vi "example_02_convert.vi"() -> ()   [LabVIEW 2015, in "lv-unit-conversion.lvlib"] (continued)
, "dimension"="M/L3", "is_si_unit"=TRUE, "category"="derived", "base_unit"="kg/m3", "conversion_reference"="DERIVED", "is_exact"=TRUE, "a"=0.0, "b"=0.45359237, "c"=158.987294928, "d"=0.0, "underlying_def"="", "description"=""}, {"symbol"="0.001 lbm/gal[UK]", "name"="pound-mass per thousand UK gallon", "dimension"="M/L3", "is_si_unit"=TRUE, "category"="derived", "base_unit"="kg/m3", "conversion_reference"="DERIVED", "is_exact"=TRUE, "a"=0.0, "b"=0.45359237, "c"=4.54609, "d"=0.0, "underlying_def"="", "description"=""}, {"symbol"="0.001 lbm/gal[US]", "name"="pound-mass per thousand US gallon", "dimension"="M/L3", "is_si_unit"=TRUE, "category"="derived", "base_unit"="kg/m3", "conversion_reference"="DERIVED", "is_exact"=TRUE, "a"=0.0, "b"=0.45359237, "c"=3.785411784, "d"=0.0, "underlying_def"="", "description"=""}, {"symbol"="0.01 grain/ft3", "name"="grain per hundred cubic foot", "dimension"="M/L3", "is_si_unit"=TRUE, "category"="derived", "base_unit"="kg/m3", "conversion_reference"="DERIVED", "is_exact"=TRUE, "a"=0.0, "b"=6.479891e-05, "c"=2.8316846592, "d"=0.0, "underlying_def"="", "description"=""}, {"symbol"="0.1 lbm/bbl", "name"="pound-mass per ten barrel", "dimension"="M/L3", "is_si_unit"=TRUE, "category"="derived", "base_unit"="kg/m3", "conversion_reference"="DERIVED", "is_exact"=TRUE, "a"=0.0, "b"=0.45359237, "c"=1.58987294928, "d"=0.0, "underlying_def"="", "description"=""}, {"symbol"="10 Mg/m3", "name"="ten thousand kilogram per cubic metre", "dimension"="M/L3", "is_si_unit"=TRUE, "category"="derived", "base_unit"="kg/m3", "conversion_reference"="DERIVED", "is_exact"=TRUE, "a"=0.0, "b"=10000.0, "c"=1.0, "d"=0.0, "underlying_def"="", "description"=""}, {"symbol"="g/cm3", "name"="gram per cubic centimetre", "dimension"="M/L3", "is_si_unit"=TRUE, "category"="derived", "base_unit"="kg/m3", "conversion_reference"="DERIVED", "is_exact"=TRUE, "a"=0.0, "b"=1000.0, "c"=1.0, "d"=0.0, "underlying_def"="", "description"=""}, {"symbol"="g/dm3", "name"="gram per cubic decimetre", "dimension"="M/L3", "is_si_unit"=TRUE, "category"="derived", "base_unit"="kg/m3", "conversion_reference"="DERIVED", "is_exact"=TRUE, "a"=0.0, "b"=1.0, "c"=1.0, "d"=0.0, "underlying_def"="", "description"=""}, {"symbol"="g/gal[UK]", "name"="gram per UK gallon", "dimension"="M/L3", "is_si_unit"=TRUE, "category"="derived", "base_unit"="kg/m3", "conversion_reference"="DERIVED", "is_exact"=TRUE, "a"=0.0, "b"=0.001, "c"=0.00454609, "d"=0.0, "underlying_def"="", "description"=""}, {"symbol"="g/gal[US]", "name"="gram per US gallon", "dimension"="M/L3", "is_si_unit"=TRUE, "category"="derived", "base_unit"="kg/m3", "conversion_reference"="DERIVED", "is_exact"=TRUE, "a"=0.0, "b"=0.001, "c"=0.003785411784, "d"=0.0, "underlying_def"="", "description"=""}, {"symbol"="g/L", "name"="gram per litre", "dimension"="M/L3", "is_si_unit"=TRUE, "category"="derived", "base_unit"="kg/m3", "conversion_reference"="DERIVED", "is_exact"=TRUE, "a"=0.0, "b"=1.0, "c"=1.0, "d"=0.0, "underlying_def"="", "description"=""}, {"symbol"="g/m3", "name"="gram per cubic metre", "dimension"="M/L3", "is_si_unit"=TRUE, "category"="derived", "base_unit"="kg/m3", "conversion_reference"="DERIVED", "is_exact"=TRUE, "a"=0.0, "b"=0.001, "c"=1.0, "d"=0.0, "underlying_def"="", "description"=""}, {"symbol"="grain/ft3", "name"="grain per cubic foot", "dimension"="M/L3", "is_si_unit"=TRUE, "category"="derived", "base_unit"="kg/m3", "conversion_reference"="DERIVED", "is_exact"=TRUE, "a"=0.0, "b"=6.479891e-05, "c"=0.028316846592, "d"=0.0, "underlying_def"="", "description"=""}, {"symbol"="grain/gal[US]", "name"="grain per US gallon", "dimension"="M/L3", "is_si_unit"=TRUE, "category"="derived", "base_unit"="kg/m3", "conversion_reference"="DERIVED", "is_exact"=TRUE, "a"=0.0, "b"=6.479891e-05, "c"=0.003785411784, "d"=0.0, "underlying_def"="", "description"=""}, {"symbol"="kg/dm3", "name"="kilogram per cubic decimetre", "dimension"="M/L3", "is_si_unit"=TRUE, "category"="derived", "base_unit"="kg/m3", "conversion_reference"="DERIVED", "is_exact"=TRUE, "a"=0.0, "b"=1000.0, "c"=1.0, "d"=0.0, "underlying_def"="", "description"=""}, {"symbol"="kg/L", "name"="kilogram per litre", "dimension"="M/L3", "is_si_unit"=TRUE, "category"="derived", "base_unit"="kg/m3", "conversion_reference"="DERIVED", "is_exact"=TRUE, "a"=0.0, "b"=1000.0, "c"=1.0, "d"=0.0, "underlying_def"="", "description"=""}, {"symbol"="lbm/bbl", "name"="pound-mass per barrel", "dimension"="M/L3", "is_si_unit"=TRUE, "category"="derived", "base_unit"="kg/m3", "conversion_reference"="DERIVED", "is_exact"=TRUE, "a"=0.0, "b"=0.45359237, "c"=0.158987294928, "d"=0.0, "underlying_def"="", "description"=""}, {"symbol"="lbm/ft3", "name"="pound-mass per cubic foot", "dimension"="M/L3", "is_si_unit"=TRUE, "category"="derived", "base_unit"="kg/m3", "conversion_reference"="DERIVED", "is_exact"=TRUE, "a"=0.0, "b"=0.45359237, "c"=0.028316846592, "d"=0.0, "underlying_def"="", "description"=""}, {"symbol"="lbm/gal[UK]", "name"="pound-mass per UK gallon", "dimension"="M/L3", "is_si_unit"=TRUE, "category"="derived", "base_unit"="kg/m3", "conversion_reference"="DERIVED", "is_exact"=TRUE, "a"=0.0, "b"=0.45359237, "c"=0.00454609, "d"=0.0, "underlying_def"="", "description"=""}, {"symbol"="lbm/gal[US]", "name"="pound-mass per US gallon", "dimension"="M/L3", "is_si_unit"=TRUE, "category"="derived", "base_unit"="kg/m3", "conversion_reference"="DERIVED", "is_exact"=TRUE, "a"=0.0, "b"=0.45359237, "c"=0.003785411784, "d"=0.0, "underlying_def"="", "description"=""}, {"symbol"="lbm/in3", "name"="pound-mass per cubic inch", "dimension"="M/L3", "is_si_unit"=TRUE, "category"="derived", "base_unit"="kg/m3", "conversion_reference"="DERIVED", "is_exact"=TRUE, "a"=0.0, "b"=0.45359237, "c"=1.6387064e-05, "d"=0.0, "underlying_def"="", "description"=""}, {"symbol"="mg/dm3", "name"="milligram per cubic decimetre", "dimension"="M/L3", "is_si_unit"=TRUE, "category"="derived", "base_unit"="kg/m3", "conversion_reference"="DERIVED", "is_exact"=TRUE, "a"=0.0, "b"=0.001, "c"=1.0, "d"=0.0, "underlying_def"="", "description"=""}, {"symbol"="mg/gal[US]", "name"="milligram per US gallon", "dimension"="M/L3", "is_si_unit"=TRUE, "category"="derived", "base_unit"="kg/m3", "conversion_reference"="DERIVED", "is_exact"=TRUE, "a"=0.0, "b"=1e-06, "c"=0.003785411784, "d"=0.0, "underlying_def"="", "description"=""}, {"symbol"="mg/L", "name"="milligram per litre", "dimension"="M/L3", "is_si_unit"=TRUE, "category"="derived", "base_unit"="kg/m3", "conversion_reference"="DERIVED", "is_exact"=TRUE, "a"=0.0, "b"=0.001, "c"=1.0, "d"=0.0, "underlying_def"="", "description"=""}, {"symbol"="Mg/m3", "name"="megagram per cubic metre", "dimension"="M/L3", "is_si_unit"=TRUE, "category"="derived", "base_unit"="kg/m3", "conversion_reference"="DERIVED", "is_exact"=TRUE, "a"=0.0, "b"=1000.0, "c"=1.0, "d"=0.0, "underlying_def"="", "description"=""}, {"symbol"="mg/m3", "name"="milligram per cubic metre", "dimension"="M/L3", "is_si_unit"=TRUE, "category"="derived", "base_unit"="kg/m3", "conversion_reference"="DERIVED", "is_exact"=TRUE, "a"=0.0, "b"=1e-06, "c"=1.0, "d"=0.0, "underlying_def"="", "description"=""}, {"symbol"="t/m3", "name"="tonne per cubic metre", "dimension"="M/L3", "is_si_unit"=TRUE, "category"="derived", "base_unit"="kg/m3", "conversion_reference"="DERIVED", "is_exact"=TRUE, "a"=0.0, "b"=1000.0, "c"=1.0, "d"=0.0, "underlying_def"="", "description"=""}, {"symbol"="ug/cm3", "name"="microgram per cubic centimetre", "dimension"="M/L3", "is_si_unit"=TRUE, "category"="derived", "base_unit"="kg/m3", "conversion_reference"="DERIVED", "is_exact"=TRUE, "a"=0.0, "b"=0.001, "c"=1.0, "d"=0.0, "underlying_def"="", "description"=""}, {"symbol"="kg/m4", "name"="kilogram per metre to the fourth power", "dimension"="M/L4", "is_si_unit"=TRUE, "category"="derived", "base_unit"="", "conversion_reference"="", "is_exact"=FALSE, "a"=0.0, "b"=0.0, "c"=0.0, "d"=0.0, "underlying_def"="", "description"=""}, {"symbol"="g/cm4", "name"="gram per centimetre to the fourth power", "dimension"="M/L4", "is_si_unit"=TRUE, "category"="derived", "base_unit"="kg/m4", "conversion_reference"="DERIVED", "is_exact"=TRUE, "a"=0.0, "b"=100000.0, "c"=1.0, "d"=0.0, "underlying_def"="", "description"=""}, {"symbol"="kg/dm4", "name"="kilogram per decimetre to the fourth power", "dimension"="M/L4", "is_si_unit"=TRUE, "category"="derived", "base_unit"="kg/m4", "conversion_reference"="DERIVED", "is_exact"=TRUE, "a"=0.0, "b"=10000.0, "c"=1.0, "d"=0.0, "underlying_def"="", "description"=""}, {"symbol"="lbm/(gal[UK].ft)", "name"="pound-mass per UK gallon foot", "dimension"="M/L4", "is_si_unit"=TRUE, "category"="derived", "base_unit"="kg/m4", "conversion_reference"="DERIVED", "is_exact"=TRUE, "a"=0.0, "b"=0.45359237, "c"=0.001385648232, "d"=0.0, "underlying_def"="", "description"=""}, {"symbol"="lbm/(gal[US].ft)", "name"="pound-mass per US gallon foot", "dimension"="M/L4", "is_si_unit"=TRUE, "category"="derived", "base_unit"="kg/m4", "conversion_reference"="DERIVED", "is_exact"=TRUE, "a"=0.0, "b"=0.45359237, "c"=0.0011537935117632, "d"=0.0, "underlying_def"="", "description"=""}, {"symbol"="lbm/ft4", "name"="pound-mass per foot to the fourth power", "dimension"="M/L4", "is_si_unit"=TRUE, "category"="derived", "base_unit"="kg/m4", "conversion_reference"="DERIVED", "is_exact"=TRUE, "a"=0.0, "b"=0.45359237, "c"=0.0086309748412416, "d"=0.0, "underlying_def"="", "description"=""}, {"symbol"="Pa.s2/m3", "name"="pascal second squared per cubic metre", "dimension"="M/L4", "is_si_unit"=TRUE, "category"="derived", "base_unit"="kg/m4", "conversion_reference"="DERIVED", "is_exact"=TRUE, "a"=0.0, "b"=1.0, "c"=1.0, "d"=0.0, "underlying_def"="", "description"=""}, {"symbol"="Pa.s/m3", "name"="pascal second per cubic metre", "dimension"="M/L4T", "is_si_unit"=TRUE, "category"="derived", "base_unit"="", "conversion_reference"="", "is_exact"=FALSE, "a"=0.0, "b"=0.0, "c"=0.0, "d"=0.0, "underlying_def"="", "description"=""}, {"symbol"="psi.d/bbl", "name"="psi day per barrel", "dimension"="M/L4T", "is_si_unit"=TRUE, "category"="derived", "base_unit"="Pa.s/m3", "conversion_reference"="DERIVED", "is_exact"=TRUE, "a"=0.0, "b"=384326.3475585072, "c"=0.00010257224319574849, "d"=0.0, "underlying_def"="", "description"=""}, {"symbol"="Pa/m3", "name"="pascal per cubic metre", "dimension"="M/L4T2", "is_si_unit"=TRUE, "category"="derived", "base_unit"="", "conversion_reference"="", "is_exact"=FALSE, "a"=0.0, "b"=0.0, "c"=0.0, "d"=0.0, "underlying_def"="", "description"=""}, {"symbol"="psi2.d/(cP.ft3)", "name"="psi squared day per centipoise cubic foot", "dimension"="M/L4T2", "is_si_unit"=TRUE, "category"="derived", "base_unit"="Pa/m3", "conversion_reference"="DERIVED", "is_exact"=TRUE, "a"=0.0, "b"=1709568766.5238712, "c"=1.1786361425484662e-08, "d"=0.0, "underlying_def"="", "description"=""}, {"symbol"="P", "name"="poise", "dimension"="M/LT", "is_si_unit"=TRUE, "category"="atom", "base_unit"="Pa.s", "conversion_reference"="NIST-SI", "is_exact"=TRUE, "a"=0.0, "b"=0.1, "c"=1.0, "d"=0.0, "underlying_def"="dyne.s/cm2", "description"="The poise is the CGS unit for viscosity (also called dynamic viscosity)."}, {"symbol"="kg/(m.s)", "name"="kilogram per metre second", "dimension"="M/LT", "is_si_unit"=TRUE, "category"="derived", "base_unit"="", "conversion_reference"="", "is_exact"=FALSE, "a"=0.0, "b"=0.0, "c"=0.0, "d"=0.0, "underlying_def"="Pa.s", "description"=""}, {"symbol"="Pa.s", "name"="pascal second", "dimension"="M/LT", "is_si_unit"=TRUE, "category"="derived", "base_unit"="", "conversion_reference"="", "is_exact"=FALSE, "a"=0.0, "b"=0.0, "c"=0.0, "d"=0.0, "underlying_def"="", "description"=""}, {"symbol"="lbm/(ft.h)", "name"="pound-mass per hour foot", "dimension"="M/LT", "is_si_unit"=TRUE, "category"="derived", "base_unit"="kg/(m.s)", "conversion_reference"="DERIVED", "is_exact"=TRUE, "a"=0.0, "b"=0.45359237, "c"=1097.28, "d"=0.0, "underlying_def"="", "description"=""}, {"symbol"="lbm/(ft.s)", "name"="pound-mass per second foot", "dimension"="M/LT", "is_si_unit"=TRUE, "category"="derived", "base_unit"="kg/(m.s)", "conversion_reference"="DERIVED", "is_exact"=TRUE, "a"=0.0, "b"=0.45359237, "c"=0.3048, "d"=0.0, "underlying_def"="", "description"=""}, {"symbol"="dyne.s/cm2", "name"="dyne second per square centimetre", "dimension"="M/LT", "is_si_unit"=TRUE, "category"="derived", "base_unit"="Pa.s", "conversion_reference"="DERIVED", "is_exact"=TRUE, "a"=0.0, "b"=0.1, "c"=1.0, "d"=0.0, "underlying_def"="", "description"=""}, {"symbol"="kgf.s/m2", "name"="thousand gram-force second per square metre", "dimension"="M/LT", "is_si_unit"=TRUE, "category"="derived", "base_unit"="Pa.s", "conversion_reference"="DERIVED", "is_exact"=TRUE, "a"=0.0, "b"=9.80665, "c"=1.0, "d"=0.0, "underlying_def"="", "description"=""}, {"symbol"="lbf.s/ft2", "name"="pound-force second per square foot", "dimension"="M/LT", "is_si_unit"=TRUE, "category"="derived", "base_unit"="Pa.s", "conversion_reference"="DERIVED", "is_exact"=TRUE, "a"=0.0, "b"=4.4482216152605, "c"=0.09290304, "d"=0.0, "underlying_def"="", "description"=""}, {"symbol"="lbf.s/in2", "name"="pound-force second per square inch", "dimension"="M/LT", "is_si_unit"=TRUE, "category"="derived", "base_unit"="Pa.s", "conversion_reference"="DERIVED", "is_exact"=TRUE, "a"=0.0, "b"=4.4482216152605, "c"=0.00064516, "d"=0.0, "underlying_def"="", "description"=""}, {"symbol"="mPa.s", "name"="millipascal second", "dimension"="M/LT", "is_si_unit"=TRUE, "category"="derived", "base_unit"="Pa.s", "conversion_reference"="DERIVED", "is_exact"=TRUE, "a"=0.0, "b"=0.001, "c"=1.0, "d"=0.0, "underlying_def"="", "description"=""}, {"symbol"="N.s/m2", "name"="newton second per square metre", "dimension"="M/LT", "is_si_unit"=TRUE, "category"="derived", "base_unit"="Pa.s", "conversion_reference"="DERIVED", "is_exact"=TRUE, "a"=0.0, "b"=1.0, "c"=1.0, "d"=0.0, "underlying_def"="", "description"=""}, {"symbol"="psi.s", "name"="psi second", "dimension"="M/LT", "is_si_unit"=TRUE, "category"="derived", "base_unit"="Pa.s", "conversion_reference"="DERIVED", "is_exact"=TRUE, "a"=0.0, "b"=4.4482216152605, "c"=0.00064516, "d"=0.0, "underlying_def"="", "description"=""}, {"symbol"="cP", "name"="centipoise", "dimension"="M/LT", "is_si_unit"=TRUE, "category"="prefixed", "base_unit"="Pa.s", "conversion_reference"="DERIVED", "is_exact"=TRUE, "a"=0.0, "b"=0.001, "c"=1.0, "d"=0.0, "underlying_def"="", "description"=""}, {"symbol"="dP", "name"="decipoise", "dimension"="M/LT", "is_si_unit"=TRUE, "category"="prefixed", "base_unit"="Pa.s", "conversion_reference"="DERIVED", "is_exact"=TRUE, "a"=0.0, "b"=0.01, "c"=1.0, "d"=0.0, "underlying_def"="", "description"=""}, {"symbol"="EP", "name"="exapoise", "dimension"="M/LT", "is_si_unit"=TRUE, "category"="prefixed", "base_unit"="Pa.s", "conversion_reference"="DERIVED", "is_exact"=TRUE, "a"=0.0, "b"=1e+17, "c"=1.0, "d"=0.0, "underlying_def"="", "description"=""}, {"symbol"="fP", "name"="femtopoise", "dimension"="M/LT", "is_si_unit"=TRUE, "category"="prefixed", "base_unit"="Pa.s", "conversion_reference"="DERIVED", "is_exact"=TRUE, "a"=0.0, "b"=1e-16, "c"=1.0, "d"=0.0, "underlying_def"="", "description"=""}, {"symbol"="GP", "name"="gigapoise", "dimension"="M/LT", "is_si_unit"=TRUE, "category"="prefixed", "base_unit"="Pa.s", "conversion_reference"="DERIVED", "is_exact"=TRUE, "a"=0.0, "b"=100000000.0, "c"=1.0, "d"=0.0, "underlying_def"="", "description"=""}, {"symbol"="kP", "name"="kilopoise", "dimension"="M/LT", "is_si_unit"=TRUE, "category"="prefixed", "base_unit"="Pa.s", "conversion_reference"="DERIVED", "is_exact"=TRUE, "a"=0.0, "b"=100.0, "c"=1.0, "d"=0.0, "underlying_def"="", "description"=""}, {"symbol"="mP", "name"="millipoise", "dimension"="M/LT", "is_si_unit"=TRUE, "category"="prefixed", "base_unit"="Pa.s", "conversion_reference"="DERIVED", "is_exact"=TRUE, "a"=0.0, "b"=0.0001, "c"=1.0, "d"=0.0, "underlying_def"="", "description"=""}, {"symbol"="MP", "name"="megapoise", "dimension"="M/LT", "is_si_unit"=TRUE, "category"="prefixed", "base_unit"="Pa.s", "conversion_reference"="DERIVED", "is_exact"=TRUE, "a"=0.0, "b"=100000.0, "c"=1.0, "d"=0.0, "underlying_def"="", "description"=""}, {"symbol"="nP", "name"="nanopoise", "dimension"="M/LT", "is_si_unit"=TRUE, "category"="prefixed", "base_unit"="Pa.s", "conversion_reference"="DERIVED", "is_exact"=TRUE, "a"=0.0, "b"=1e-10, "c"=1.0, "d"=0.0, "underlying_def"="", "description"=""}, {"symbol"="pP", "name"="picopoise", "dimension"="M/LT", "is_si_unit"=TRUE, "category"="prefixed", "base_unit"="Pa.s", "conversion_reference"="DERIVED", "is_exact"=TRUE, "a"=0.0, "b"=1e-13, "c"=1.0, "d"=0.0, "underlying_def"="", "description"=""}, {"symbol"="TP", "name"="terapoise", "dimension"="M/LT", "is_si_unit"=TRUE, "category"="prefixed", "base_unit"="Pa.s", "conversion_reference"="DERIVED", "is_exact"=TRUE, "a"=0.0, "b"=100000000000.0, "c"=1.0, "d"=0.0, "underlying_def"="", "description"=""}, {"symbol"="uP", "name"="micropoise", "dimension"="M/LT", "is_si_unit"=TRUE, "category"="prefixed", "base_unit"="Pa.s", "conversion_reference"="DERIVED", "is_exact"=TRUE, "a"=0.0, "b"=1e-07, "c"=1.0, "d"=0.0, "underlying_def"="", "description"=""}, {"symbol"="Pa", "name"="pascal", "dimension"="M/LT2", "is_si_unit"=TRUE, "category"="atom-special", "base_unit"="", "conversion_reference"="", "is_exact"=FALSE, "a"=0.0, "b"=0.0, "c"=0.0, "d"=0.0, "underlying_def"="J/m3", "description"="The pressure or stress of 1 N/m2."}, {"symbol"="at", "name"="technical atmosphere", "dimension"="M/LT2", "is_si_unit"=TRUE, "category"="atom", "base_unit"="Pa", "conversion_reference"="NIST-SI", "is_exact"=TRUE, "a"=0.0, "b"=98066.5, "c"=1.0, "d"=0.0, "underlying_def"="kgf/cm2", "description"="One technical atmosphere equals one kilogram-force per square centimeter (1 at = 1 kgf/cm2). \n\t\t\t\tFrom NIST.\n\t\t\t"}, {"symbol"="atm", "name"="standard atmosphere", "dimension"="M/LT2", "is_si_unit"=TRUE, "category"="atom", "base_unit"="Pa", "conversion_reference"="NIST-SI", "is_exact"=TRUE, "a"=0.0, "b"=101325.0, "c"=1.0, "d"=0.0, "underlying_def"="101.325 kPa", "description"="An international reference pressure defined as 101.325 kPa and formerly used as unit of pressure. \n\t\t\t\tFor practical purposes it has been replaced by the bar which is 100 kPa. \n\t\t\t\tThe difference of about 1% is not significant for many applications, and is within the error range \n\t\t\t\tof common pressure gauges.\n\t\t\t"}, {"symbol"="bar", "name"="bar", "dimension"="M/LT2", "is_si_unit"=TRUE, "category"="atom-allowed", "base_unit"="Pa", "conversion_reference"="NIST-SI", "is_exact"=TRUE, "a"=0.0, "b"=100000.0, "c"=1.0, "d"=0.0, "underlying_def"="100 kPa", "description"="100 kPa. \n\t\t\t\tSince 1982 one bar has been used as the standard pressure for tabulating all thermodynamic data. \n\t\t\t\tPrior to 1982 the standard pressure used to be the standard atmosphere, equal to 1.013 25 bar, or \n\t\t\t\t101 325 Pa.\n\t\t\t"}, {"symbol"="cmH2O[4degC]", "name"="centimetre of water at 4 degree Celsius", "dimension"="M/LT2", "is_si_unit"=TRUE, "category"="atom", "base_unit"="Pa", "conversion_reference"="NIST-SI", "is_exact"=TRUE, "a"=0.0, "b"=98.0638, "c"=1.0, "d"=0.0, "underlying_def"="", "description"="NIST-SI gives a limited number of digits of precision and states the following: \"Additional digits \n\t\t\t\tare not justified because the definitions of the units do not take into account the compressibility \n\t\t\t\tof mercury or the change in density caused by the revised practical temperature scale, ITS-90. \n\t\t\t\tSimilar comments also apply to water manometer pressure units.\"\n\t\t\t"}, {"symbol"="inH2O[39degF]", "name"="inch of water at 39.2 degree Fahrenheit", "dimension"="M/LT2", "is_si_unit"=TRUE, "category"="atom", "base_unit"="Pa", "conversion_reference"="NIST-SI", "is_exact"=TRUE, "a"=0.0, "b"=249.082, "c"=1.0, "d"=0.0, "underlying_def"="", "description"="NIST-SI gives a limited number of digits of precision and states the following: \"Additional digits \n\t\t\t\tare not justified because the definitions of the units do not take into account the compressibility \n\t\t\t\tof mercury or the change in density caused by the revised practical temperature scale, ITS-90. \n\t\t\t\tSimilar comments also apply to water manometer pressure units.\"\n\t\t\t"}, {"symbol"="inH2O[60degF]", "name"="inch of water at 60 degree Fahrenheit", "dimension"="M/LT2", "is_si_unit"=TRUE, "category"="atom", "base_unit"="Pa", "conversion_reference"="NIST-SI", "is_exact"=TRUE, "a"=0.0, "b"=248.84, "c"=1.0, "d"=0.0, "underlying_def"="", "description"="NIST-SI gives a limited number of digits of precision and states the following: \"Additional digits \n\t\t\t\tare not justified because the definitions of the units do not take into account the compressibility \n\t\t\t\tof mercury or the change in density caused by the revised practical temperature scale, ITS-90. \n\t\t\t\tSimilar comments also apply to water manometer pressure units.\"\n\t\t\t"}, {"symbol"="inHg[32degF]", "name"="inch of mercury at 32 degree Fahrenheit", "dimension"="M/LT2", "is_si_unit"=TRUE, "category"="atom", "base_unit"="Pa", "conversion_reference"="NIST-SI", "is_exact"=TRUE, "a"=0.0, "b"=3386.38, "c"=1.0, "d"=0.0, "underlying_def"="", "description"="NIST-SI gives a limited number of digits of precision and states the following: \"Additional digits \n\t\t\t\tare not justified because the definitions of the units do not take into account the compressibility \n\t\t\t\tof mercury or the change in density caused by the revised practical temperature scale, ITS-90. \n\t\t\t\tSimilar comments also apply to water manometer pressure units.\"\n\t\t\t"}, {"symbol"="inHg[60degF]", "name"="inch of mercury at 60 degree Fahrenheit", "dimension"="M/LT2", "is_si_unit"=TRUE, "category"="atom", "base_unit"="Pa", "conversion_reference"="NIST-SI", "is_exact"=TRUE, "a"=0.0, "b"=3376.85, "c"=1.0, "d"=0.0, "underlying_def"="", "description"="NIST-SI gives a limited number of digits of precision and states the following: \"Additional digits \n\t\t\t\tare not justified because the definitions of the units do not take into account the compressibility \n\t\t\t\tof mercury or the change in density caused by the revised practical temperature scale, ITS-90. \n\t\t\t\tSimilar comments also apply to water manometer pressure units.\"\n\t\t\t"}, {"symbol"="mmHg[0degC]", "name"="millimetres of Mercury at 0 deg C", "dimension"="M/LT2", "is_si_unit"=TRUE, "category"="atom", "base_unit"="Pa", "conversion_reference"="NIST-SI", "is_exact"=TRUE, "a"=0.0, "b"=133.322, "c"=1.0, "d"=0.0, "underlying_def"="", "description"="NIST-SI gives a limited number of digits of precision and states the following: \"Additional digits \n\t\t\t\tare not justified because the definitions of the units do not take into account the compressibility \n\t\t\t\tof mercury or the change in density caused by the revised practical temperature scale, ITS-90. \n\t\t\t\tSimilar comments also apply to water manometer pressure units.\"\n\t\t\t"}, {"symbol"="psi", "name"="pound-force per square inch", "dimension"="M/LT2", "is_si_unit"=TRUE, "category"="atom-special", "base_unit"="Pa", "conversion_reference"="DEFINITION", "is_exact"=TRUE, "a"=0.0, "b"=4.4482216152605, "c"=0.00064516, "d"=0.0, "underlying_def"="lbf/in2", "description"="Pound-force per square inch. \n\t\t\t\tA unit of pressure or of stress based on avoirdupois units. \n\t\t\t\tIt is the pressure resulting from a force of one pound-force applied to an area of one square inch.\n\t\t\t"}, {"symbol"="torr", "name"="torr", "dimension"="M/LT2", "is_si_unit"=TRUE, "category"="atom", "base_unit"="Pa", "conversion_reference"="NIST-SI", "is_exact"=TRUE, "a"=0.0, "b"=101325.0, "c"=760.0, "d"=0.0, "underlying_def"="1/760 atm", "description"="The torr is defined as 1/760 of one atmosphere, while the atmosphere is defined as 101.325 kPa. \n\t\t\t\tTherefore, 1 Torr is equal to 101325/760 Pa (from Wikipedia).\n\t\t\t"}, {"symbol"="umHg[0degC]", "name"="micrometre of mercury at 0 degree Celsius", "dimension"="M/LT2", "is_si_unit"=TRUE, "category"="atom", "base_unit"="Pa", "conversion_reference"="NIST-SI", "is_exact"=TRUE, "a"=0.0, "b"=0.133322, "c"=1.0, "d"=0.0, "underlying_def"="", "description"="NIST-SI gives a limited number of digits of precision and states the following: \"Additional digits \n\t\t\t\tare not justified because the definitions of the units do not take into account the compressibility \n\t\t\t\tof mercury or the change in density caused by the revised practical temperature scale, ITS-90. \n\t\t\t\tSimilar comments also apply to water manometer pressure units.\"\n\t\t\t"}, {"symbol"="J/m3", "name"="joule per cubic metre", "dimension"="M/LT2", "is_si_unit"=TRUE, "category"="derived", "base_unit"="", "conversion_reference"="", "is_exact"=FALSE, "a"=0.0, "b"=0.0, "c"=0.0, "d"=0.0, "underlying_def"="", "description"=""}, {"symbol"="Btu[IT]/bbl", "name"="BTU per barrel", "dimension"="M/LT2", "is_si_unit"=TRUE, "category"="derived", "base_unit"="J/m3", "conversion_reference"="DERIVED", "is_exact"=TRUE, "a"=0.0, "b"=1055.05585262, "c"=0.158987294928, "d"=0.0, "underlying_def"="", "description"=""}, {"symbol"="Btu[IT]/ft3", "name"="BTU per cubic foot", "dimension"="M/LT2", "is_si_unit"=TRUE, "category"="derived", "base_unit"="J/m3", "conversion_reference"="DERIVED", "is_exact"=TRUE, "a"=0.0, "b"=1055.05585262, "c"=0.028316846592, "d"=0.0, "underlying_def"="", "description"=""}, {"symbol"="Btu[IT]/gal[UK]", "name"="BTU per UK gallon", "dimension"="M/LT2", "is_si_unit"=TRUE, "category"="derived", "base_unit"="J/m3", "conversion_reference"="DERIVED", "is_exact"=TRUE, "a"=0.0, "b"=1055.05585262, "c"=0.00454609, "d"=0.0, "underlying_def"="", "description"=""}, {"symbol"="Btu[IT]/gal[US]", "name"="BTU per US gallon", "dimension"="M/LT2", "is_si_unit"=TRUE, "category"="derived", "base_unit"="J/m3", "conversion_reference"="DERIVED", "is_exact"=TRUE, "a"=0.0, "b"=1055.05585262, "c"=0.003785411784, "d"=0.0, "underlying_def"="", "description"=""}, {"symbol"="cal[th]/cm3", "name"="calorie per cubic centimetre", "dimension"="M/LT2", "is_si_unit"=TRUE, "category"="derived", "base_unit"="J/m3", "conversion_reference"="DERIVED", "is_exact"=TRUE, "a"=0.0, "b"=4184000.0, "c"=1.0, "d"=0.0, "underlying_def"="", "description"=""}, {"symbol"="cal[th]/mL", "name"="calorie per millilitre", "dimension"="M/LT2", "is_si_unit"=TRUE, "category"="derived", "base_unit"="J/m3", "conversion_reference"="DERIVED", "is_exact"=TRUE, "a"=0.0, "b"=4184000.0, "c"=1.0, "d"=0.0, "underlying_def"="", "description"=""}, {"symbol"="cal[th]/mm3", "name"="calorie per cubic millimetre", "dimension"="M/LT2", "is_si_unit"=TRUE, "category"="derived", "base_unit"="J/m3", "conversion_reference"="DERIVED", "is_exact"=TRUE, "a"=0.0, "b"=4184000000.0, "c"=1.0, "d"=0.0, "underlying_def"="", "description"=""}, {"symbol"="erg/cm3", "name"="erg per cubic centimetre", "dimension"="M/LT2", "is_si_unit"=TRUE, "category"="derived", "base_unit"="J/m3", "conversion_reference"="DERIVED", "is_exact"=TRUE, "a"=0.0, "b"=0.1, "c"=1.0, "d"=0.0, "underlying_def"="", "description"=""}, {"symbol"="erg/m3", "name"="erg per cubic metre", "dimension"="M/LT2", "is_si_unit"=TRUE, "category"="derived", "base_unit"="J/m3", "conversion_reference"="DERIVED", "is_exact"=TRUE, "a"=0.0, "b"=1e-07, "c"=1.0, "d"=0.0, "underlying_def"="", "description"=""}, {"symbol"="hp.h/bbl", "name"="horsepower hour per barrel", "dimension"="M/LT2", "is_si_unit"=TRUE, "category"="derived", "base_unit"="J/m3", "conversion_reference"="DERIVED", "is_exact"=TRUE, "a"=0.0, "b"=2684519.537696173, "c"=0.158987294928, "d"=0.0, "underlying_def"="", "description"=""}, {"symbol"="J/dm3", "name"="joule per cubic decimetre", "dimension"="M/LT2", "is_si_unit"=TRUE, "category"="derived", "base_unit"="J/m3", "conversion_reference"="DERIVED", "is_exact"=TRUE, "a"=0.0, "b"=1000.0, "c"=1.0, "d"=0.0, "underlying_def"="", "description"=""}, {"symbol"="kcal[th]/cm3", "name"="thousand calorie per cubic centimetre", "dimension"="M/LT2", "is_si_unit"=TRUE, "category"="derived", "base_unit"="J/m3", "conversion_reference"="DERIVED", "is_exact"=TRUE, "a"=0.0, "b"=4184000000.0, "c"=1.0, "d"=0.0, "underlying_def"="", "description"=""}, {"symbol"="kcal[th]/m3", "name"="thousand calorie per cubic metre", "dimension"="M/LT2", "is_si_unit"=TRUE, "category"="derived", "base_unit"="J/m3", "conversion_reference"="DERIVED", "is_exact"=TRUE, "a"=0.0, "b"=4184.0, "c"=1.0, "d"=0.0, "underlying_def"="", "description"=""}, {"symbol"="kJ/dm3", "name"="kilojoule per cubic decimetre", "dimension"="M/LT2", "is_si_unit"=TRUE, "category"="derived", "base_unit"="J/m3", "conversion_reference"="DERIVED", "is_exact"=TRUE, "a"=0.0, "b"=1000000.0, "c"=1.0, "d"=0.0, "underlying_def"="", "description"=""}, {"symbol"="kJ/m3", "name"="kilojoule per cubic metre", "dimension"="M/LT2", "is_si_unit"=TRUE, "category"="derived", "base_unit"="J/m3", "conversion_reference"="DERIVED", "is_exact"=TRUE, "a"=0.0, "b"=1000.0, "c"=1.0, "d"=0.0, "underlying_def"="", "description"=""}, {"symbol"="kW.h/dm3", "name"="kilowatt hour per cubic decimetre", "dimension"="M/LT2", "is_si_unit"=TRUE, "category"="derived", "base_unit"="J/m3", "conversion_reference"="DERIVED", "is_exact"=TRUE, "a"=0.0, "b"=3600000000.0, "c"=1.0, "d"=0.0, "underlying_def"="", "description"=""}, {"symbol"="kW.h/m3", "name"="kilowatt hour per cubic metre", "dimension"="M/LT2", "is_si_unit"=TRUE, "category"="derived", "base_unit"="J/m3", "conversion_reference"="DERIVED", "is_exact"=TRUE, "a"=0.0, "b"=3600000.0, "c"=1.0, "d"=0.0, "underlying_def"="", "description"=""}, {"symbol"="lbf.ft/bbl", "name"="foot pound-force per barrel", "dimension"="M/LT2", "is_si_unit"=TRUE, "category"="derived", "base_unit"="J/m3", "conversion_reference"="DERIVED", "is_exact"=TRUE, "a"=0.0, "b"=1.3558179483314003, "c"=0.158987294928, "d"=0.0, "underlying_def"="", "description"=""}, {"symbol"="lbf.ft/gal[US]", "name"="foot pound-force per US gallon", "dimension"="M/LT2", "is_si_unit"=TRUE, "category"="derived", "base_unit"="J/m3", "conversion_reference"="DERIVED", "is_exact"=TRUE, "a"=0.0, "b"=1.3558179483314003, "c"=0.003785411784, "d"=0.0, "underlying_def"="", "description"=""}, {"symbol"="MJ/m3", "name"="megajoule per cubic metre", "dimension"="M/LT2", "is_si_unit"=TRUE, "category"="derived", "base_unit"="J/m3", "conversion_reference"="DERIVED", "is_exact"=TRUE, "a"=0.0, "b"=1000000.0, "c"=1.0, "d"=0.0, "underlying_def"="", "description"=""}, {"symbol"="MW.h/m3", "name"="megawatt hour per cubic metre", "dimension"="M/LT2", "is_si_unit"=TRUE, "category"="derived", "base_unit"="J/m3", "conversion_reference"="DERIVED", "is_exact"=TRUE, "a"=0.0, "b"=3600000000.0, "c"=1.0, "d"=0.0, "underlying_def"="", "description"=""}, {"symbol"="tonf[US].mi/bbl", "name"="US ton-force mile per barrel", "dimension"="M/LT2", "is_si_unit"=TRUE, "category"="derived", "base_unit"="J/m3", "conversion_reference"="DERIVED", "is_exact"=TRUE, "a"=0.0, "b"=14317437.534379588, "c"=0.158987294928, "d"=0.0, "underlying_def"="", "description"=""}, {"symbol"="0.01 lbf/ft2", "name"="pound-force per hundred square foot", "dimension"="M/LT2", "is_si_unit"=TRUE, "category"="derived", "base_unit"="Pa", "conversion_reference"="DERIVED", "is_exact"=TRUE, "a"=0.0, "b"=4.4482216152605, "c"=9.290304, "d"=0.0, "underlying_def"="", "description"=""}, {"symbol"="dyne/cm2", "name"="dyne per square centimetre", "dimension"="M/LT2", "is_si_unit"=TRUE, "category"="derived", "base_unit"="Pa", "conversion_reference"="DERIVED", "is_exact"=TRUE, "a"=0.0, "b"=0.1, "c"=1.0, "d"=0.0, "underlying_def"="", "description"=""}, {"symbol"="kgf/cm2", "name"="thousand gram-force per square centimetre", "dimension"="M/LT2", "is_si_unit"=TRUE, "category"="derived", "base_unit"="Pa", "conversion_reference"="DERIVED", "is_exact"=TRUE, "a"=0.0, "b"=98066.5, "c"=1.0, "d"=0.0, "underlying_def"="", "description"=""}, {"symbol"="kgf/m2", "name"="thousand gram-force per square metre", "dimension"="M/LT2", "is_si_unit"=TRUE, "category"="derived", "base_unit"="Pa", "conversion_reference"="DERIVED", "is_exact"=TRUE, "a"=0.0, "b"=9.80665, "c"=1.0, "d"=0.0, "underlying_def"="", "description"=""}, {"symbol"="kgf/mm2", "name"="thousand gram-force per square millimetre", "dimension"="M/LT2", "is_si_unit"=TRUE, "category"="derived", "base_unit"="Pa", "conversion_reference"="DERIVED", "is_exact"=TRUE, "a"=0.0, "b"=9806650.0, "c"=1.0, "d"=0.0, "underlying_def"="", "description"=""}, {"symbol"="kN/m2", "name"="kilonewton per square metre", "dimension"="M/LT2", "is_si_unit"=TRUE, "category"="derived", "base_unit"="Pa", "conversion_reference"="DERIVED", "is_exact"=TRUE, "a"=0.0, "b"=1000.0, "c"=1.0, "d"=0.0, "underlying_def"="", "description"=""}, {"symbol"="lbf/ft2", "name"="pound-force per square foot", "dimension"="M/LT2", "is_si_unit"=TRUE, "category"="derived", "base_unit"="Pa", "conversion_reference"="DERIVED", "is_exact"=TRUE, "a"=0.0, "b"=4.4482216152605, "c"=0.09290304, "d"=0.0, "underlying_def"="", "description"=""}, {"symbol"="N/m2", "name"="newton per square metre", "dimension"="M/LT2", "is_si_unit"=TRUE, "category"="derived", "base_unit"="Pa", "conversion_reference"="DERIVED", "is_exact"=TRUE, "a"=0.0, "b"=1.0, "c"=1.0, "d"=0.0, "underlying_def"="", "description"=""}, {"symbol"="N/mm2", "name"="newton per square millimetre", "dimension"="M/LT2", "is_si_unit"=TRUE, "category"="derived", "base_unit"="Pa", "conversion_reference"="DERIVED", "is_exact"=TRUE, "a"=0.0, "b"=1000000.0, "c"=1.0, "d"=0.0, "underlying_def"="", "description"=""}, {"symbol"="tonf[UK]/ft2", "name"="UK ton-force per square foot", "dimension"="M/LT2", "is_si_unit"=TRUE, "category"="derived", "base_unit"="Pa", "conversion_reference"="DERIVED", "is_exact"=TRUE, "a"=0.0, "b"=9964.01641818352, "c"=0.09290304, "d"=0.0, "underlying_def"="", "description"=""}, {"symbol"="tonf[US]/ft2", "name"="US ton-force per square foot", "dimension"="M/LT2", "is_si_unit"=TRUE, "category"="derived", "base_unit"="Pa", "conversion_reference"="DERIVED", "is_exact"=TRUE, "a"=0.0, "b"=8896.443230521, "c"=0.09290304, "d"=0.0, "underlying_def"="", "description"=""}, {"symbol"="tonf[US]/in2", "name"="US ton-force per square inch", "dimension"="M/LT2", "is_si_unit"=TRUE, "category"="derived", "base_unit"="Pa", "conversion_reference"="DERIVED", "is_exact"=TRUE, "a"=0.0, "b"=8896.443230521, "c"=0.00064516, "d"=0.0, "underlying_def"="", "description"=""}, {"symbol"="cPa", "name"="centipascal", "dimension"="M/LT2", "is_si_unit"=TRUE, "category"="prefixed", "base_unit"="Pa", "conversion_reference"="DERIVED", "is_exact"=TRUE, "a"=0.0, "b"=0.01, "c"=1.0, "d"=0.0, "underlying_def"="", "description"=""}, {"symbol"="dPa", "name"="decipascal", "dimension"="M/LT2", "is_si_unit"=TRUE, "category"="prefixed", "base_unit"="Pa", "conversion_reference"="DERIVED", "is_exact"=TRUE, "a"=0.0, "b"=0.1, "c"=1.0, "d"=0.0, "underlying_def"="", "description"=""}, {"symbol"="EPa", "name"="exapascal", "dimension"="M/LT2", "is_si_unit"=TRUE, "category"="prefixed", "base_unit"="Pa", "conversion_reference"="DERIVED", "is_exact"=TRUE, "a"=0.0, "b"=1e+18, "c"=1.0, "d"=0.0, "underlying_def"="", "description"=""}, {"symbol"="fPa", "name"="femtopascal", "dimension"="M/LT2", "is_si_unit"=TRUE, "category"="prefixed", "base_unit"="Pa", "conversion_reference"="DERIVED", "is_exact"=TRUE, "a"=0.0, "b"=1e-15, "c"=1.0, "d"=0.0, "underlying_def"="", "description"=""}, {"symbol"="GPa", "name"="gigapascal", "dimension"="M/LT2", "is_si_unit"=TRUE, "category"="prefixed", "base_unit"="Pa", "conversion_reference"="DERIVED", "is_exact"=TRUE, "a"=0.0, "b"=1000000000.0, "c"=1.0, "d"=0.0, "underlying_def"="", "description"=""}, {"symbol"="hbar", "name"="hundred bar", "dimension"="M/LT2", "is_si_unit"=TRUE, "category"="prefixed", "base_unit"="Pa", "conversion_reference"="DERIVED", "is_exact"=TRUE, "a"=0.0, "b"=10000000.0, "c"=1.0, "d"=0.0, "underlying_def"="", "description"=""}, {"symbol"="kPa", "name"="kilopascal", "dimension"="M/LT2", "is_si_unit"=TRUE, "category"="prefixed", "base_unit"="Pa", "conversion_reference"="DERIVED", "is_exact"=TRUE, "a"=0.0, "b"=1000.0, "c"=1.0, "d"=0.0, "underlying_def"="", "description"=""}, {"symbol"="kpsi", "name"="thousand psi", "dimension"="M/LT2", "is_si_unit"=TRUE, "category"="prefixed", "base_unit"="Pa", "conversion_reference"="DERIVED", "is_exact"=TRUE, "a"=0.0, "b"=4448.2216152605, "c"=0.00064516, "d"=0.0, "underlying_def"="", "description"=""}, {"symbol"="mbar", "name"="thousandth of bar", "dimension"="M/LT2", "is_si_unit"=TRUE, "category"="prefixed", "base_unit"="Pa", "conversion_reference"="DERIVED", "is_exact"=TRUE, "a"=0.0, "b"=100.0, "c"=1.0, "d"=0.0, "underlying_def"="", "description"=""}, {"symbol"="mPa", "name"="millipascal", "dimension"="M/LT2", "is_si_unit"=TRUE, "category"="prefixed", "base_unit"="Pa", "conversion_reference"="DERIVED", "is_exact"=TRUE, "a"=0.0, "b"=0.001, "c"=1.0, "d"=0.0, "underlying_def"="", "description"=""}, {"symbol"="MPa", "name"="megapascal", "dimension"="M/LT2", "is_si_unit"=TRUE, "category"="prefixed", "base_unit"="Pa", "conversion_reference"="DERIVED", "is_exact"=TRUE, "a"=0.0, "b"=1000000.0, "c"=1.0, "d"=0.0, "underlying_def"="", "description"=""}, {"symbol"="Mpsi", "name"="million psi", "dimension"="M/LT2", "is_si_unit"=TRUE, "category"="prefixed", "base_unit"="Pa", "conversion_reference"="DERIVED", "is_exact"=TRUE, "a"=0.0, "b"=4448221.6152605, "c"=0.00064516, "d"=0.0, "underlying_def"="", "description"=""}, {"symbol"="nPa", "name"="nanopascal", "dimension"="M/LT2", "is_si_unit"=TRUE, "category"="prefixed", "base_unit"="Pa", "conversion_reference"="DERIVED", "is_exact"=TRUE, "a"=0.0, "b"=1e-09, "c"=1.0, "d"=0.0, "underlying_def"="", "description"=""}, {"symbol"="pPa", "name"="picopascal", "dimension"="M/LT2", "is_si_unit"=TRUE, "category"="prefixed", "base_unit"="Pa", "conversion_reference"="DERIVED", "is_exact"=TRUE, "a"=0.0, "b"=1e-12, "c"=1.0, "d"=0.0, "underlying_def"="", "description"=""}, {"symbol"="TPa", "name"="terapascal", "dimension"="M/LT2", "is_si_unit"=TRUE, "category"="prefixed", "base_unit"="Pa", "conversion_reference"="DERIVED", "is_exact"=TRUE, "a"=0.0, "b"=1000000000000.0, "c"=1.0, "d"=0.0, "underlying_def"="", "description"=""}, {"symbol"="ubar", "name"="millionth of bar", "dimension"="M/LT2", "is_si_unit"=TRUE, "category"="prefixed", "base_unit"="Pa", "conversion_reference"="DERIVED", "is_exact"=TRUE, "a"=0.0, "b"=0.1, "c"=1.0, "d"=0.0, "underlying_def"="", "description"=""}, {"symbol"="uPa", "name"="micropascal", "dimension"="M/LT2", "is_si_unit"=TRUE, "category"="prefixed", "base_unit"="Pa", "conversion_reference"="DERIVED", "is_exact"=TRUE, "a"=0.0, "b"=1e-06, "c"=1.0, "d"=0.0, "underlying_def"="", "description"=""}, {"symbol"="upsi", "name"="millionth of psi", "dimension"="M/LT2", "is_si_unit"=TRUE, "category"="prefixed", "base_unit"="Pa", "conversion_reference"="DERIVED", "is_exact"=TRUE, "a"=0.0, "b"=4.4482216152605e-06, "c"=0.00064516, "d"=0.0, "underlying_def"="", "description"=""}, {"symbol"="Pa/s", "name"="pascal per second", "dimension"="M/LT3", "is_si_unit"=TRUE, "category"="derived", "base_unit"="", "conversion_reference"="", "is_exact"=FALSE, "a"=0.0, "b"=0.0, "c"=0.0, "d"=0.0, "underlying_def"="W/m3", "description"=""}, {"symbol"="Pa2/(Pa.s)", "name"="pascal squared per pascal second", "dimension"="M/LT3", "is_si_unit"=TRUE, "category"="derived", "base_unit"="", "conversion_reference"="", "is_exact"=FALSE, "a"=0.0, "b"=0.0, "c"=0.0, "d"=0.0, "underlying_def"="W/m3", "description"=""}, {"symbol"="W/m3", "name"="watt per cubic metre", "dimension"="M/LT3", "is_si_unit"=TRUE, "category"="derived", "base_unit"="", "conversion_reference"="", "is_exact"=FALSE, "a"=0.0, "b"=0.0, "c"=0.0, "d"=0.0, "underlying_def"="", "description"=""}, {"symbol"="atm/h", "name"="standard atmosphere per hour", "dimension"="M/LT3", "is_si_unit"=TRUE, "category"="derived", "base_unit"="Pa/s", "conversion_reference"="DERIVED", "is_exact"=TRUE, "a"=0.0, "b"=101325.0, "c"=3600.0, "d"=0.0, "underlying_def"="", "description"=""}, 
